vi "rep_cap_remove.vi"(6 "Rep Cap Name":string, 7 "error in":errorcluster, 8 "Rep Cap Name ID":string, 10 "VISA resource name":refnum<visa-resource-name>) -> (0 "error out":errorcluster, 3 "VISA resource name out":refnum<visa-resource-name>)   [LabVIEW 2014, in "rszvl_rsidr_core.lvlib"]
uses:
  rszvl_rsidr_core.lvlib
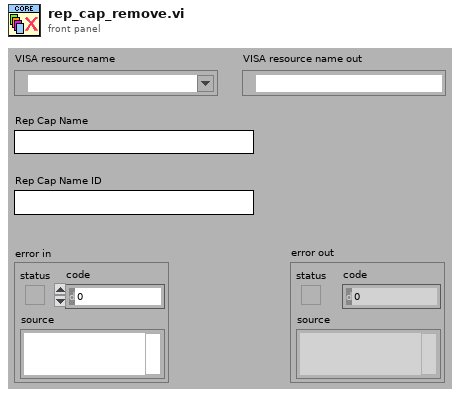
[diagram p1: front panel]
types:
  T1 = enum16{"Initialize", "Get Cmd Value", "Reset Rep Cap", "Add Rep Cap", "Remove Rep Cap", "Get Rep Cap ID range", "Get Count", "Clear", "Find Name from NameID", "Get First NameID"}
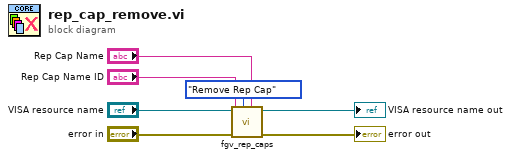
[diagram p0: block diagram]
diagram:
  n1 = call "fgv_rep_caps.vi"("RepCapName in (\"\")"="Rep Cap Name", "Operation"=T1."Remove Rep Cap", "error in"="error in", "RepCapNameID in (\"\")"="Rep Cap Name ID", "VISA resource name"="VISA resource name") -> ("error out"=→"error out":errorcluster, "VISA resource name out"=→"VISA resource name out":refnum<visa-resource-name>)  [unwired: 3 in, 2 out]
